vi "SQL Table Create and edit.vi"() -> ()   [LabVIEW 2017]
uses:
  <vilib>/addons/database/Auxilliary.llb/DB Tools Column Info.ctl
  <vilib>/addons/database/Auxilliary.llb/DB Tools DataTypes.ctl
  <vilib>/addons/database/Connection.llb/DB Tools Open Connec (Path).vi
  <vilib>/addons/database/NI_Database_API.lvlib
panel:
  in  "Delete Data Only from Table":bool
  out "error out":errorcluster
  in  "column information":T1[](array[typedef])
  in  "Table name":string
  in  "Create Table":bool
  in  "stop":bool
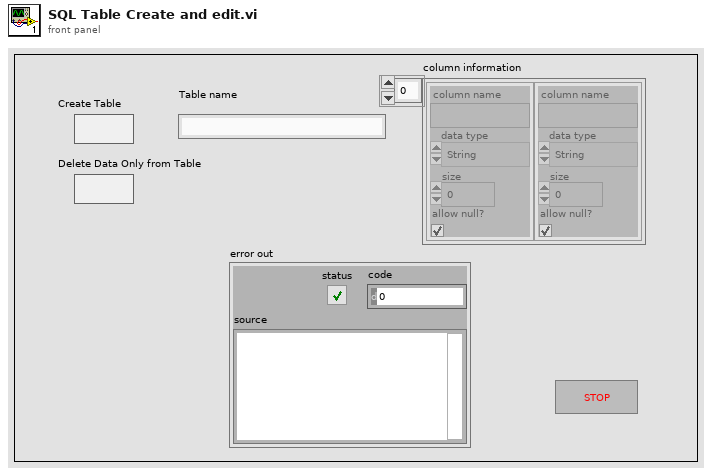
[diagram p1: front panel]
types:
  T1 = typedef "NI_Database_API.lvlib/DB Tools Column Info.ctl" = cluster{"column name":string, "data type":T2, "size":i32, "allow null?":bool}
  T2 = typedef "NI_Database_API.lvlib/DB Tools DataTypes.ctl" = enum16{"String", "Long (I32)", "Single (SGL)", "Double (DBL)", "Date/Time", "Binary"}
  T3 = typedef "NI_Database_API.lvlib/Conn ObjectReference.ctl" = refnum<k1>
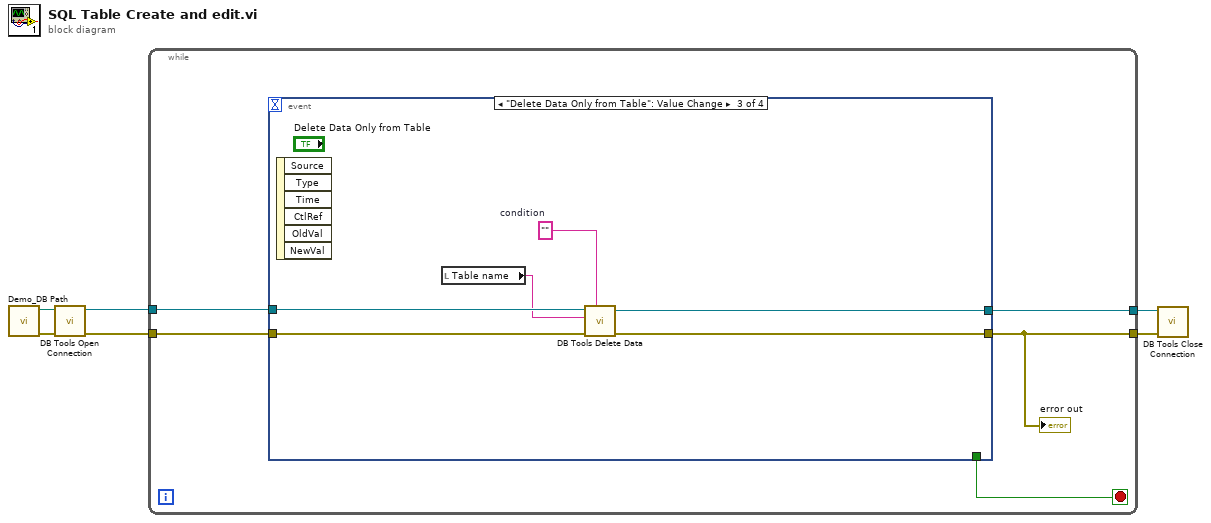
[diagram p0: block diagram]
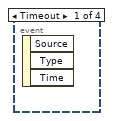
[diagram p2: hidden frame]
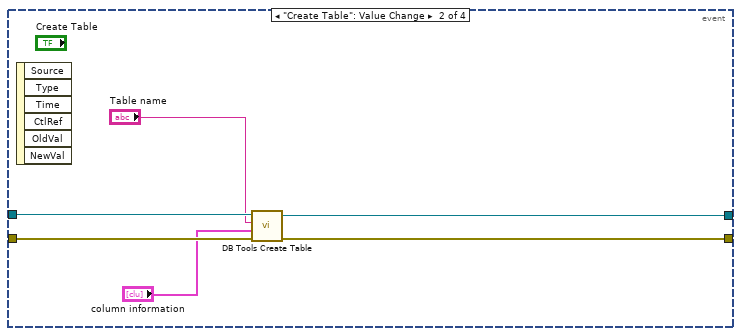
[diagram p3: hidden frame]
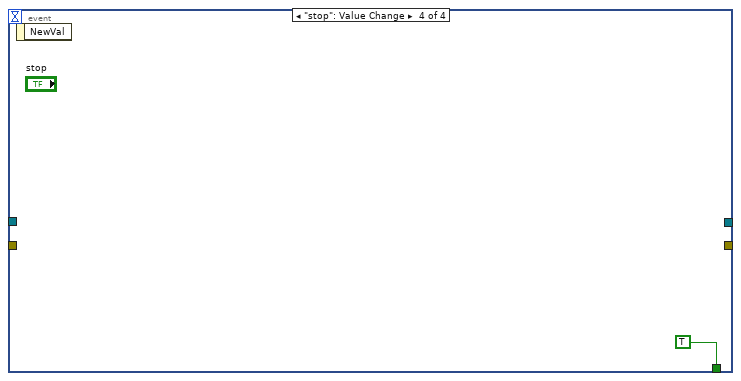
[diagram p4: hidden frame]
diagram:
  n1 = call "Demo_DB Path.vi"() -> ("error out"=w6:errorcluster, "DB Path"=w5:path)  [unwired: 10 in]
  n2 = call-poly <vilib>:"DB Tools Open Connection.vi"("error in (no error)"=w6, "connection information"=w5) -> ("error out"=w4:errorcluster, "connection reference"=w3:T3)  [unwired: 6 in]
  n3 = while {
    tunnel: w4 -> [w10]
    tunnel: w3 -> [w9]
    tunnel: [w8] -> w2
    tunnel: [w7] -> w1
    stop <- w11 stop-if-true
    n4 = event shown="[2] \"Delete Data Only from Table\": Value Change" {
      selector: _ -> [_ _ _ _]
      dyn-events: _ -> [_ _ _ _]
      timeout: _ -> [_ _ _ _]
      tunnel: [_ _ _ TRUE] -> w11
      tunnel: w10 -> [_ w16 w22 _]
      tunnel: w9 -> [_ w17 w23 _]
      tunnel: [_ w15 w21 _] -> w8
      tunnel: [_ w14 w20 _] -> w7
      event Timeout {
        n5 = event-data() -> ()  [unwired: 1 in, 3 out]
      }
      event "Create Table": Value Change {
        n6 = event-data() -> ()  [unwired: 1 in, 6 out]
        n7 = call <vilib>:"DB Tools Create Table.vi"("error in (no error)"=w16, "column information"="column information", "table"="Table name", "connection reference"=w17) -> ("error out"=w15:errorcluster, "connection reference out"=w14:T3)  [unwired: 4 in]
      }
      event "Delete Data Only from Table": Value Change {
        w18 = ""  # condition
        n8 = event-data() -> ()  [unwired: 1 in, 6 out]
        n9 = local read "Table name"() -> (w19:string)
        n10 = call <vilib>:"DB Tools Delete Data.vi"("condition"=w18, "error in (no error)"=w22, "table"=w19, "connection reference"=w23) -> ("error out"=w21:errorcluster, "connection reference out"=w20:T3)  [unwired: 6 in]
      }
      event "stop": Value Change {
        n11 = event-data() -> ()  [unwired: 1 in, 1 out]
      }
    }
    "error out" <- w8
  }
  n12 = call <vilib>:"DB Tools Close Connection.vi"("error in (no error)"=w2, "connection reference"=w1) -> ()  [unwired: 5 in, 1 out]
